vi "Add Bus Controller.vi"(8 "error in":errorcluster, 9 "BusController Config":T1={"scheduleMaxEntries"=512, "scheduleIDRef"=0, "triggerMode"=0, "eventLogOnHalt"=FALSE, "eventLogOnPause"=FALSE, "stepMode"=FALSE, "syncMode"=0, "defaultGap"=8.0, "timeout"=19.0} {"syncMode" items=["Selective", "All"]; "triggerMode" items=["None", "External", "Start"]}, 10 "name":string, 11 "1553channel ref in":refnum<k24>) -> (0 "error out":errorcluster, 2 "new busController":refnum<k24>, 3 "1553channel ref out":refnum<k24>)   [LabVIEW 2020, in "Ballard_1553_Hardware_ni.lvlib"]
uses:
  Ballard_1553_Hardware_ni.lvlib
  C:/Users/Administrator/Desktop/GIT/Ballard-MIL-STD-1553-Custom-Device/Source/System Explorer/SubVIs/Parse XML Ballard/1.2/BTIXML_SerDes.dll
  Ballard-MIL-STD-1553-Custom-Device/Source/System Explorer/SubVIs/Parse XML Ballard/1.2/BTIXML_SerDes.dll
  _typedefs/BusController_type.ctl
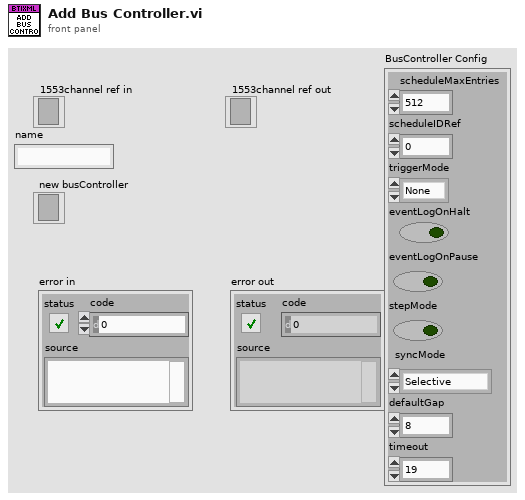
[diagram p1: front panel]
types:
  T1 = typedef "BusController_type.ctl" = cluster{"scheduleMaxEntries":u32, "scheduleIDRef":i32, "triggerMode":i32, "eventLogOnHalt":bool, "eventLogOnPause":bool, "stepMode":bool, "syncMode":i32, "defaultGap":dbl, "timeout":dbl}
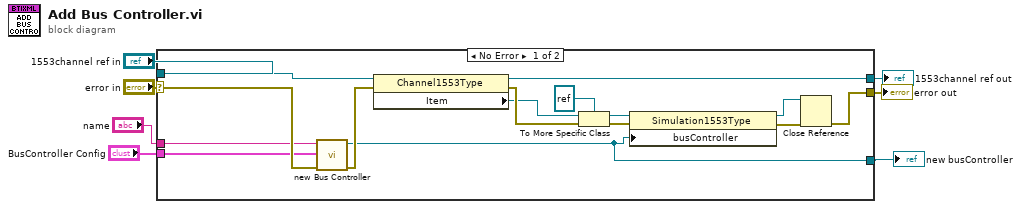
[diagram p0: block diagram]
diagram:
  n1 = case shown="No Error" "error in" {
    selector: "error in" -> [w12 w23]
    tunnel: [w13 w23] -> w7
    tunnel: [w22 w24] -> w6
    tunnel: "1553channel ref in" -> [w21 w24]
    tunnel: [w10 _] -> w3
    tunnel: "name" -> [w9 _]
    tunnel: "BusController Config" -> [w8 _]
    frame No Error {
      n2 = call "new Bus Controller.vi"("error in"=w12, "BusController Config"=w8, "name"=w9) -> ("error out"=w11:errorcluster, "xml ref out"=w10:refnum<k24>)  [unwired: 7 in]
      n3 = property class="Channel1553Type"(reference=w21, error in=w11) -> (reference out=w22:refnum<k24>, error out=w20:errorcluster, "Item"=w19:refnum<k24>)
      n4 = To More Specific Class(target class=refnum<k24> refnum, reference=w19, error in=w20) -> (specific class reference=w17:refnum<k24>, error out=w16:errorcluster)
      n5 = property class="Simulation1553Type"(reference=w17, error in=w16, "busController"=w10) -> (reference out=w14:refnum<k24>, error out=w15:errorcluster)
      n6 = Close Reference(reference=w14, error in (no error)=w15) -> (error out=w13:errorcluster)
    }
    frame Error {
    }
  }
  "error out" <- w7
  "1553channel ref out" <- w6
  "new busController" <- w3
